vi "Read VariableGroupRingRef.vi"(8 "error in (no error)":errorcluster, 11 "VMUI in":refnum<class "VMUI.lvclass">) -> (0 "error out":errorcluster, 2 "VariableGroupRingRef":refnum<vi>, 3 "VMUI out":refnum<class "VMUI.lvclass">)   [LabVIEW 2013, in "VMUI.lvclass"]
uses:
  VMUI.lvclass
  VMUI.lvclass/VMUI.ctl
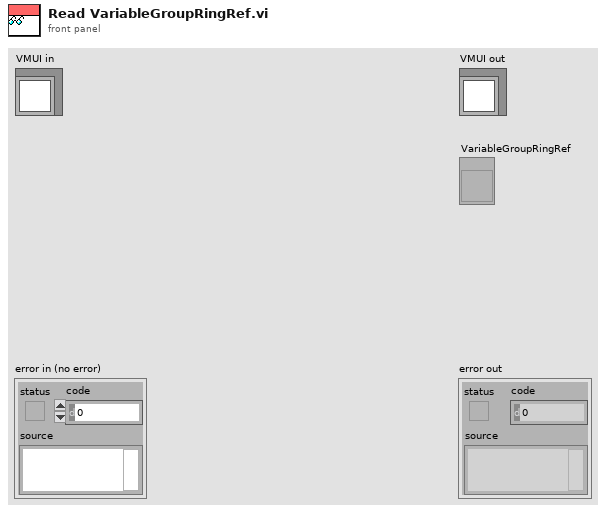
[diagram p1: front panel]
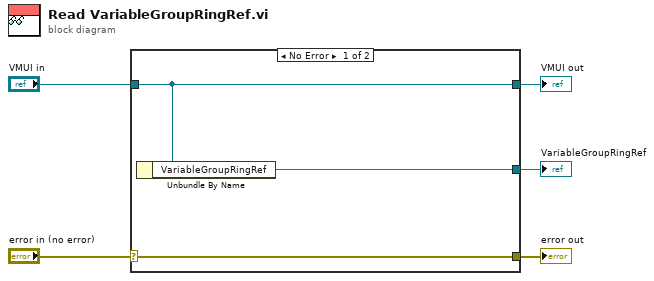
[diagram p0: block diagram]
diagram:
  n1 = case shown="No Error" "error in (no error)" {
    selector: "error in (no error)" -> [w8 w9]
    tunnel: [w8 w9] -> w4
    tunnel: [w7 w10] -> w2
    tunnel: "VMUI in" -> [w7 w10]
    tunnel: [w6 _] -> w1
    frame No Error {
      n2 = Unbundle By Name(w7) -> ("VariableGroupRingRef"=w6:refnum<vi>)
    }
    frame Error {
    }
  }
  "error out" <- w4
  "VMUI out" <- w2
  "VariableGroupRingRef" <- w1
